vi "Empty buffer.vi"(8 "Error In":errorcluster, 9 "byte count":u32=1024, 10 "Short Timeout Value":u32=200, 11 "VISA resource name":refnum<visa-resource-name>) -> (0 "Error Out":errorcluster, 2 "Buffer content":string[](array[string]), 3 "VISA resource name out":refnum<visa-resource-name>)   [LabVIEW 2019]
panel:
  out "Cycle error":errorcluster
  out "Cycle count":i32
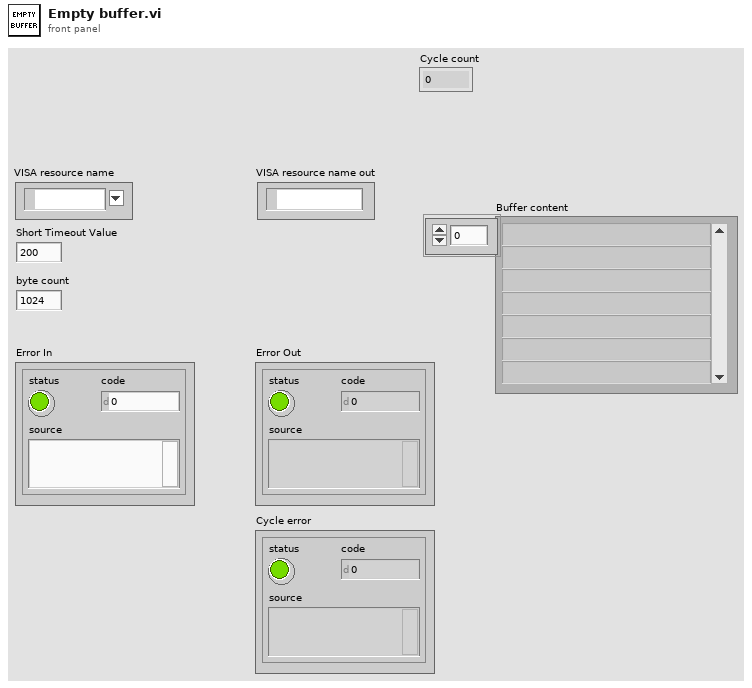
[diagram p1: front panel]
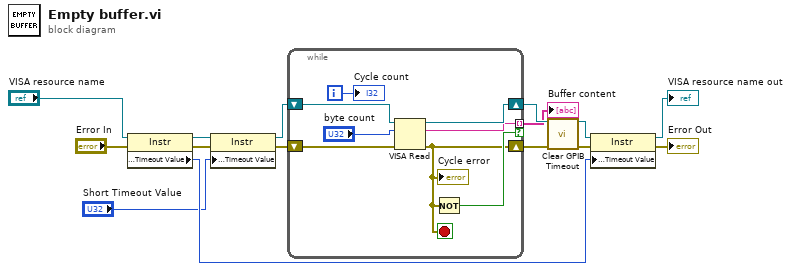
[diagram p0: block diagram]
diagram:
  n1 = property class="Instr"(reference="VISA resource name", error in="Error In") -> (reference out=w13:refnum<visa-resource-name>, error out=w12:errorcluster, "General Settings:Timeout Value"=w5:u32)
  n2 = property class="Instr"(reference=w13, error in=w12, "General Settings:Timeout Value"="Short Timeout Value") -> (reference out=w9:refnum<visa-resource-name>, error out=w10:errorcluster)
  n3 = while {
    shift-right: [w21] -> w8
    shift-left: w9 -> [w22]
    shift-right: [w15] -> w7
    shift-left: w10 -> [w20]
    tunnel: [w18] -> w1 mode=indexing if=w17
    i -> [w16]
    stop <- w15 stop-if-true
    n4 = VISA Read(VISA resource name=w22, byte count="byte count", error in (no error)=w20) -> (VISA resource name out=w21:refnum<visa-resource-name>, read buffer=w18:string, error out=w15:errorcluster)  [unwired: 1 out]
    "Cycle error" <- w15
    n5 = Not(x=w15) -> (.not. x?=w17:bool)
    "Cycle count" <- w16
  }
  "Buffer content" <- w1
  n6 = call "Clear GPIB Timeout.vi"("error in (no error)"=w7) -> ("error out"=w6:errorcluster)  [unwired: 1 in, 9 out]
  n7 = property class="Instr"(reference=w8, error in=w6, "General Settings:Timeout Value"=w5) -> (reference out=→"VISA resource name out":refnum<visa-resource-name>, error out=→"Error Out":errorcluster)
